vi "reorderPath.vi"(8 "error in (no error)":errorcluster, 11 "Array in":string[](array[string])) -> (0 "error out":errorcluster, 3 "Array out":string[](array[string]))   [LabVIEW 2015, in "Zen Analytics.lvclass"]
uses:
  Zen Analytics.lvclass
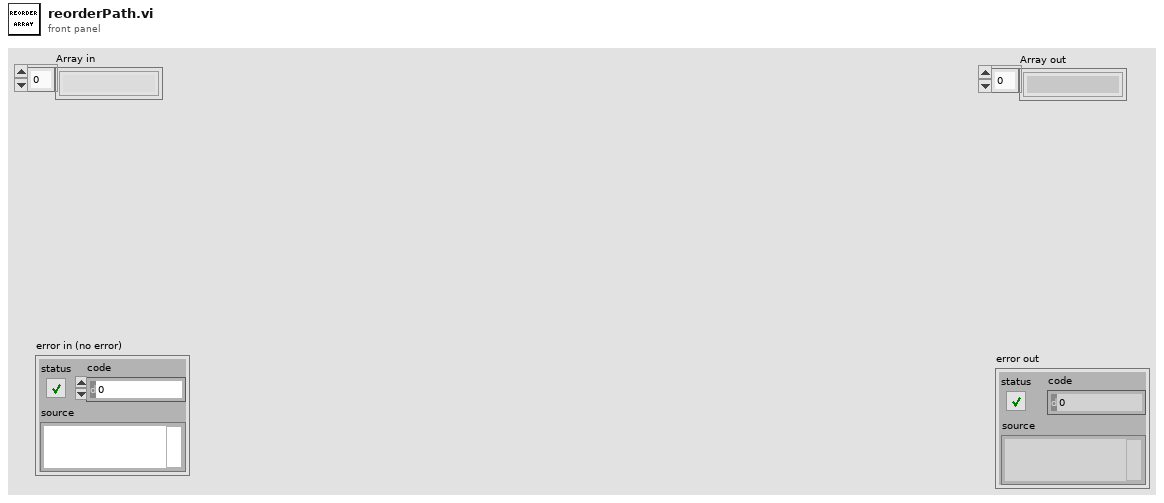
[diagram p1: front panel]
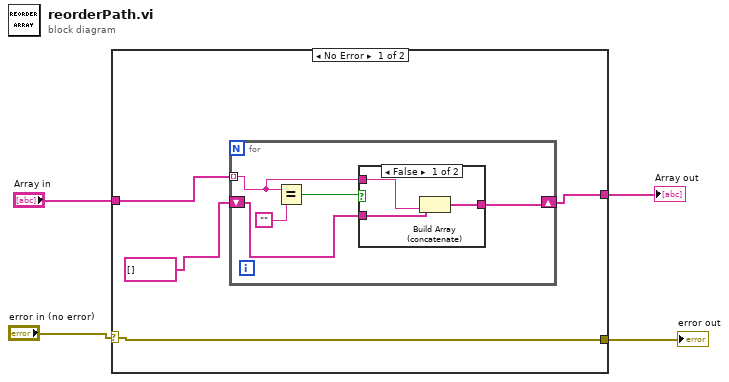
[diagram p0: block diagram]
diagram:
  n1 = case shown="No Error" "error in (no error)" {
    selector: "error in (no error)" -> [w6 w18]
    tunnel: "Array in" -> [w8 w19]
    tunnel: [w7 w19] -> w3
    tunnel: [w6 w18] -> w1
    frame No Error {
      n2 = for {
        tunnel: w8 -> [w11] mode=indexing
        shift-right: [w10] -> w7
        shift-left: string[] [] ("Array in") -> [w9]
        n3 = Equal?(x=w11, y="") -> (x = y?=w12:bool)
        n4 = case shown="False" w12 {
          tunnel: w11 -> [w16 _]
          tunnel: [w15 w17] -> w10
          tunnel: w9 -> [w14 w17]
          frame False {
            n5 = Build Array (concatenate)(w14, w16) -> (w15:string[])
          }
          frame True {
          }
        }
      }
    }
    frame Error {
    }
  }
  "Array out" <- w3
  "error out" <- w1
